vi "Get StStt.vi"(11 "N":u32) -> (2 "St":u32, 3 "Stt":u32)   [LabVIEW 2014]
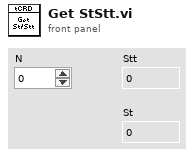
[diagram p1: front panel]
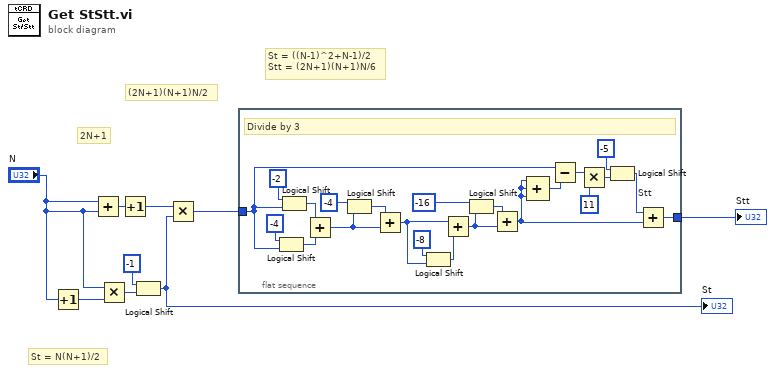
[diagram p0: block diagram]
diagram:
  # "2N+1"
  # "(2N+1)(N+1)N/2"
  # "St = N(N+1)/2"
  # "St = ((N-1)^2+N-1)/2\nStt = (2N+1)(N+1)N/6"
  n1 = Increment(x="N") -> (x+1=w6:u32)
  n2 = Add(x="N", y="N") -> (x+y=w8:u32)
  n3 = Multiply(x="N", y=w6) -> (x*y=w4:u32)
  n4 = Increment(x=w8) -> (x+1=w3:u32)
  n5 = Logical Shift(y=i16 -1, x=w4) -> (x << y=w2:u32)
  "St" <- w2
  n6 = Multiply(x=w3, y=w2) -> (x*y=w1:u32)
  n7 = flat-sequence {
    tunnel: [w11] -> w9
    tunnel: w1 -> [w10]
    frame #0 {
      # "Divide by 3"
      n8 = Logical Shift(y=i16 -4, x=w10) -> (x << y=w29:u32)
      n9 = Logical Shift(y=i16 -2, x=w10) -> (x << y=w28:u32)
      n10 = Add(x=w28, y=w29) -> (x+y=w25:u32)
      n11 = Logical Shift(y=i16 -4, x=w25) -> (x << y=w26:u32)
      n12 = Add(x=w26, y=w25) -> (x+y=w22:u32)
      n13 = Logical Shift(y=i16 -8, x=w22) -> (x << y=w23:u32)
      n14 = Add(x=w22, y=w23) -> (x+y=w19:u32)
      n15 = Logical Shift(y=i16 -16, x=w19) -> (x << y=w20:u32)
      n16 = Add(x=w20, y=w19) -> (x+y=w13:u32)
      n17 = Compound Arithmetic op=ADD(w13, w13, w13) -> (w18:u32)
      n18 = Subtract(x=w10, y=w18) -> (x-y=w17:u32)
      n19 = Multiply(x=w17, y=u32 11) -> (x*y=w15:u32)
      n20 = Logical Shift(y=i16 -5, x=w15) -> (x << y=w14:u32)
      n21 = Add "Stt"(x=w14, y=w13) -> (x+y=w11:u32)
    }
  }
  "Stt" <- w9
